vi "LVOOP Top Level.vi"() -> ()   [LabVIEW 2019]
uses:
  Command/Application Command.lvclass
  DMM/DMM.lvclass
  Initialize Command/Initialize.lvclass
  D:/Users/Marco Yang/Downloads/LVOOP 2012/LVOOP 2012/Command/Application Command.lvclass
  Initialize Command/Initialize.lvclass/Initialize.ctl
  Exit Command/Exit.lvclass
  Init DMM Command/Init DMM.lvclass
  Read/Read DMM.lvclass
  Close Command/Close DMM.lvclass
  Reset Command/Reset DMM.lvclass
panel:
  in  "Reset DMM":bool
  out "Data":dbl
  in  "Close DMM":bool
  in  "Read DMM":bool
  in  "Init DMM":bool
  in  "Stop Button":bool
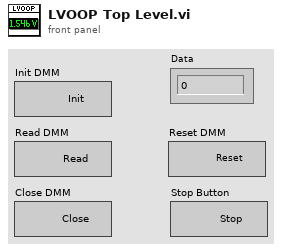
[diagram p1: front panel]
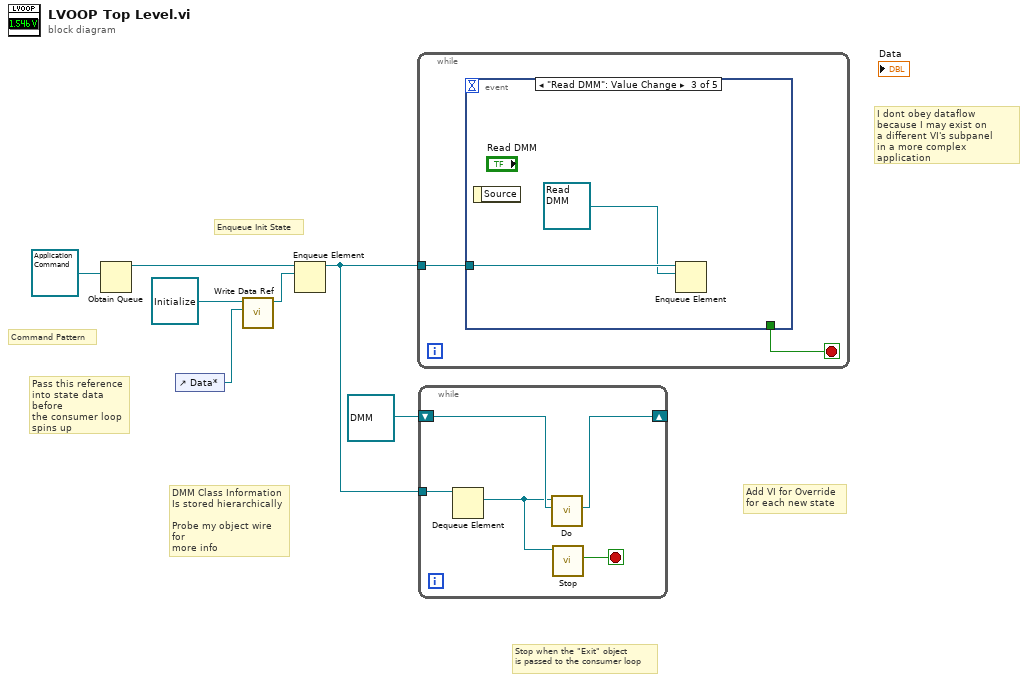
[diagram p0: block diagram]
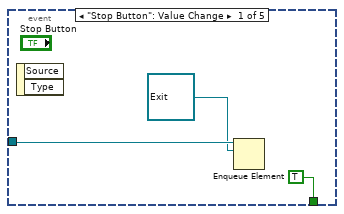
[diagram p2: hidden frame]
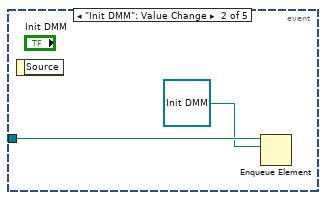
[diagram p3: hidden frame]
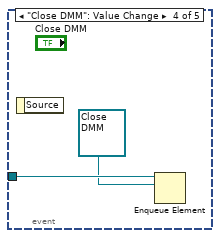
[diagram p4: hidden frame]
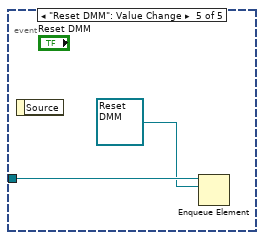
[diagram p5: hidden frame]
diagram:
  # "Enqueue Init State"
  # "DMM Class Information\nIs stored hierarchically\n\nProbe my object wire for\nmore info"
  # "Stop when the \"Exit\" object\nis passed to the consumer loop"
  # "Add VI for Override \nfor each new state"
  # "Pass this reference\ninto state data before\nthe consumer loop\nspins up"
  # "I dont obey dataflow\nbecause I may exist on\na different VI's subpanel\nin a more complex application"
  # "Command Pattern"
  n1 = Obtain Queue(element data type=refnum<class "Application Command.lvclass"> refnum ("Application Command.lvclass")) -> (queue out=w6:refnum<queue>)  [unwired: 4 in, 2 out]
  n2 = control-ref of="Data*"() -> (w1:refnum<vi>)
  n3 = call "Write Data Ref.vi"("Data*"=w1, "Initialize in"=refnum<class "Initialize.lvclass"> refnum ("Initialize.lvclass")) -> ("Initialize out"=w2:refnum<class "Initialize.lvclass">)  [unwired: 8 in, 1 out]
  n4 = Enqueue Element(queue=w6, element=w2) -> (queue out=w5:refnum<queue>)  [unwired: 2 in, 2 out]
  n5 = while {
    tunnel: w5 -> [w9]
    stop <- w8 stop-if-true
    n6 = event shown="[2] \"Read DMM\": Value Change" {
      selector: _ -> [_ _ _ _ _]
      dyn-events: _ -> [_ _ _ _ _]
      timeout: _ -> [_ _ _ _ _]
      tunnel: w9 -> [w11 w14 w16 w18 w20]
      tunnel: [TRUE _ _ _ _] -> w8
      event "Stop Button": Value Change {
        n7 = event-data() -> ()  [unwired: 1 in, 2 out]
        n8 = Enqueue Element(queue=w11, element=refnum<class "Exit.lvclass"> refnum ("Exit.lvclass")) -> ()  [unwired: 2 in, 3 out]
      }
      event "Init DMM": Value Change {
        n9 = event-data() -> ()  [unwired: 1 in, 1 out]
        n10 = Enqueue Element(queue=w14, element=refnum<class "Init DMM.lvclass"> refnum ("Init DMM.lvclass")) -> ()  [unwired: 2 in, 3 out]
      }
      event "Read DMM": Value Change {
        n11 = event-data() -> ()  [unwired: 1 in, 1 out]
        n12 = Enqueue Element(queue=w16, element=refnum<class "Read DMM.lvclass"> refnum ("Read DMM.lvclass")) -> ()  [unwired: 2 in, 3 out]
      }
      event "Close DMM": Value Change {
        n13 = event-data() -> ()  [unwired: 1 in, 1 out]
        n14 = Enqueue Element(queue=w18, element=refnum<class "Close DMM.lvclass"> refnum ("Close DMM.lvclass")) -> ()  [unwired: 2 in, 3 out]
      }
      event "Reset DMM": Value Change {
        n15 = event-data() -> ()  [unwired: 1 in, 1 out]
        n16 = Enqueue Element(queue=w20, element=refnum<class "Reset DMM.lvclass"> refnum ("Reset DMM.lvclass")) -> ()  [unwired: 2 in, 3 out]
      }
    }
  }
  n17 = while {
    tunnel: w5 -> [w25]
    shift-right: [w23] -> _
    shift-left: refnum<class "DMM.lvclass"> refnum ("DMM.lvclass") -> [w24]
    stop <- w21 stop-if-true
    n18 = Dequeue Element(queue=w25) -> (element=w22:refnum<class "Application Command.lvclass">)  [unwired: 2 in, 3 out]
    n19 = call-dynamic "Do.vi"("DMM"=w24, "Application Command in"=w22) -> ("DMM"=w23:refnum<class "DMM.lvclass">)  [unwired: 7 in, 2 out]
    n20 = call-dynamic "Stop.vi"("Application Command in"=w22) -> ("Stop"=w21:bool)  [unwired: 8 in, 2 out]
  }
